vi "Auto Calibrate.vi"(8 "error in (no error)":errorcluster, 11 "DPO4104 in":refnum<class "DPO4104.lvclass">) -> (0 "error out":errorcluster, 2 "Cal Passed ? (T:Yes)":bool, 3 "DPO4104 out":refnum<class "DPO4104.lvclass">)   [LabVIEW 2018, in "DPO4104.lvlib" / "DPO4104.lvclass"]
doc: "This Override method is used to call the Auto-Calibrate function of the Oscope instrument. The boolean output 'Cal Passed? (T:Yes)' carries out the auto-calibration result."
uses:
  DPO4104.lvclass
  PPLs/Oscilloscope/Parent/Oscilloscope.lvlibp/Oscilloscope.lvclass
  C:/Projects/LabVIEW/PPLs/Oscilloscope/Parent/Oscilloscope.lvlibp/Oscilloscope.lvclass
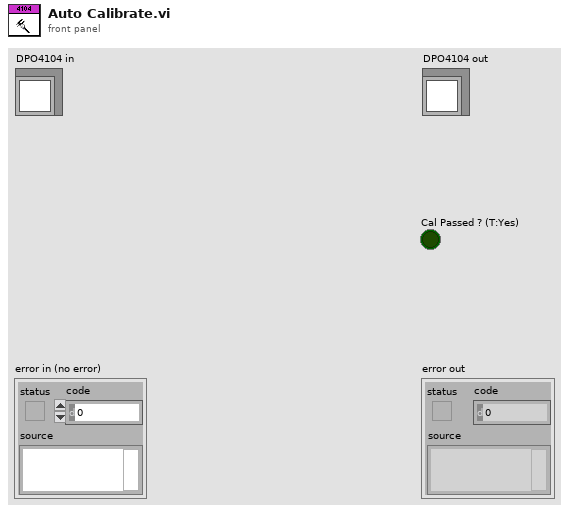
[diagram p1: front panel]
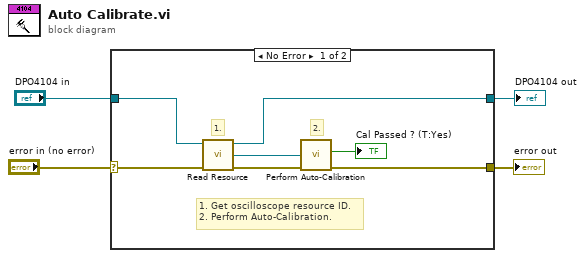
[diagram p0: block diagram]
diagram:
  n1 = case shown="No Error" "error in (no error)" {
    selector: "error in (no error)" -> [w9 w12]
    tunnel: "DPO4104 in" -> [w11 w13]
    tunnel: [w10 w13] -> w2
    tunnel: [w6 w12] -> w1
    frame No Error {
      # "1. Get oscilloscope resource ID.\n2. Perform Auto-Calibration."
      # "2."
      # "1."
      n2 = call "Read Resource.vi"("error in (no error)"=w9, "Oscilloscope in"=w11) -> ("error out"=w7:errorcluster, "Resource"=w8:refnum<visa-resource-name>, "Oscilloscope out"=w10:refnum<class "DPO4104.lvclass">)  [unwired: 7 in]
      n3 = call "Perform Auto-Calibration.vi"("error in (no error)"=w7, "VISA resource name"=w8) -> ("error out"=w6:errorcluster, "Auto-Cal Passed?"=→"Cal Passed ? (T:Yes)":bool)  [unwired: 7 in, 1 out]
    }
    frame Error {
    }
  }
  "error out" <- w1
  "DPO4104 out" <- w2
